vi "SSFG_sharp_Backup(Working).vi"() -> ()   [LabVIEW 2014]
uses:
  SSFG_States.ctl
  <vilib>/DAQmx/write.llb/DAQmx Write (Analog Wfm 1Chan NSamp).vi
  <vilib>/DAQmx/create/channels.llb/DAQmx Create Channel (AO-Voltage-Basic).vi
  <vilib>/DAQmx/configure/timing.llb/DAQmx Timing (Sample Clock).vi
  <vilib>/DAQmx/miscellaneous.llb/DAQmx Fill In Error Info.vi
  <resource>/objmgr/daqmx.rc
  <vilib>/measure/NI_MABase.lvlib
panel:
  in  "Attenuation":dbl
  out "Current State":string
  in  "Number of Samples/Cycle":dbl
  out "Waveform Graph":waveform(dbl)(graph)
  in  "stop":bool
  in  "Power Signal Parameters":T1={"Waveform Type"=0, "Amplitude"=1.0, "Frequency"=17.0} {"Frequency" format="%0.2p"; "Amplitude" scale=0.0..5.0; "Waveform Type" items=["Sine Wave", "Triangle Wave", "Square Wave", "Sawtooth Wave"]}
  out "Flicker":bool
  out "Swell":bool
  out "Sag":bool
  in  "Stop":bool
  in  "Update Rate":dbl=1000.0 format="%0.2f"
  in  "Physical Channel":tag
  in  "Flicker":T2
  in  "Swell":cluster{"Swell_Time (sec)":dbl, "Swell":bool}
  in  "Sag":cluster{"Sag_Time (sec)":dbl, "Sag":bool}
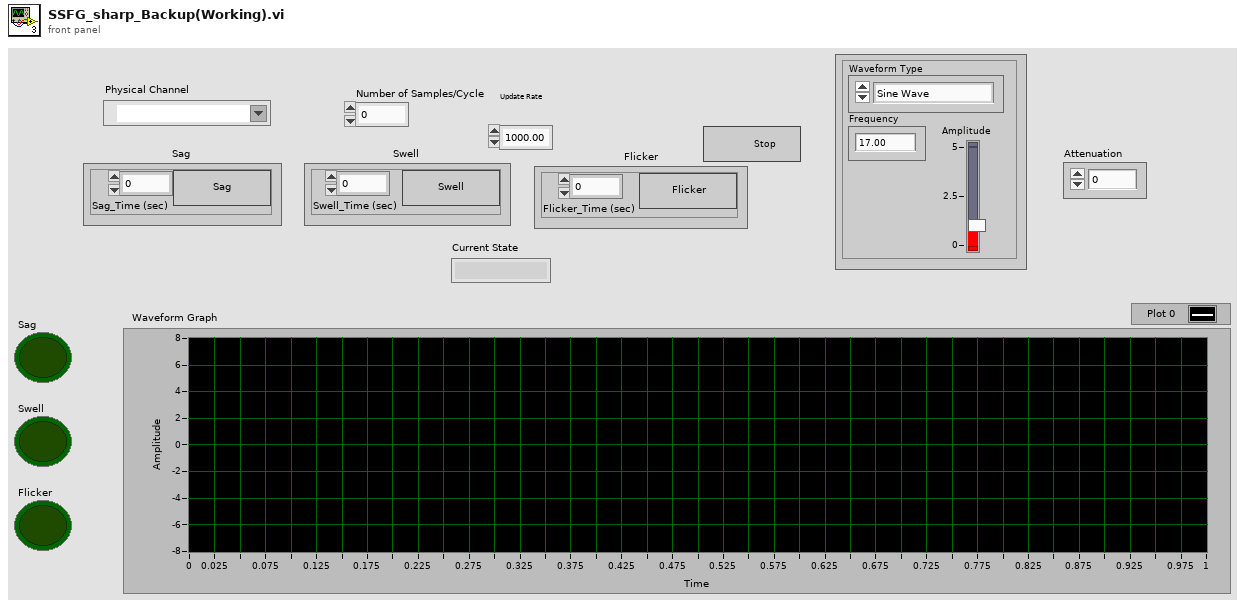
[diagram p1: front panel]
types:
  T1 = cluster{"Waveform Type":u16, "Amplitude":dbl, "Frequency":dbl}
  T2 = cluster{"Flicker_Time (sec)":dbl, "Flicker":bool}
  T3 = typedef "SSFG_States.ctl" = cluster{"State":string, "Disturbance_Time (sec)":dbl}
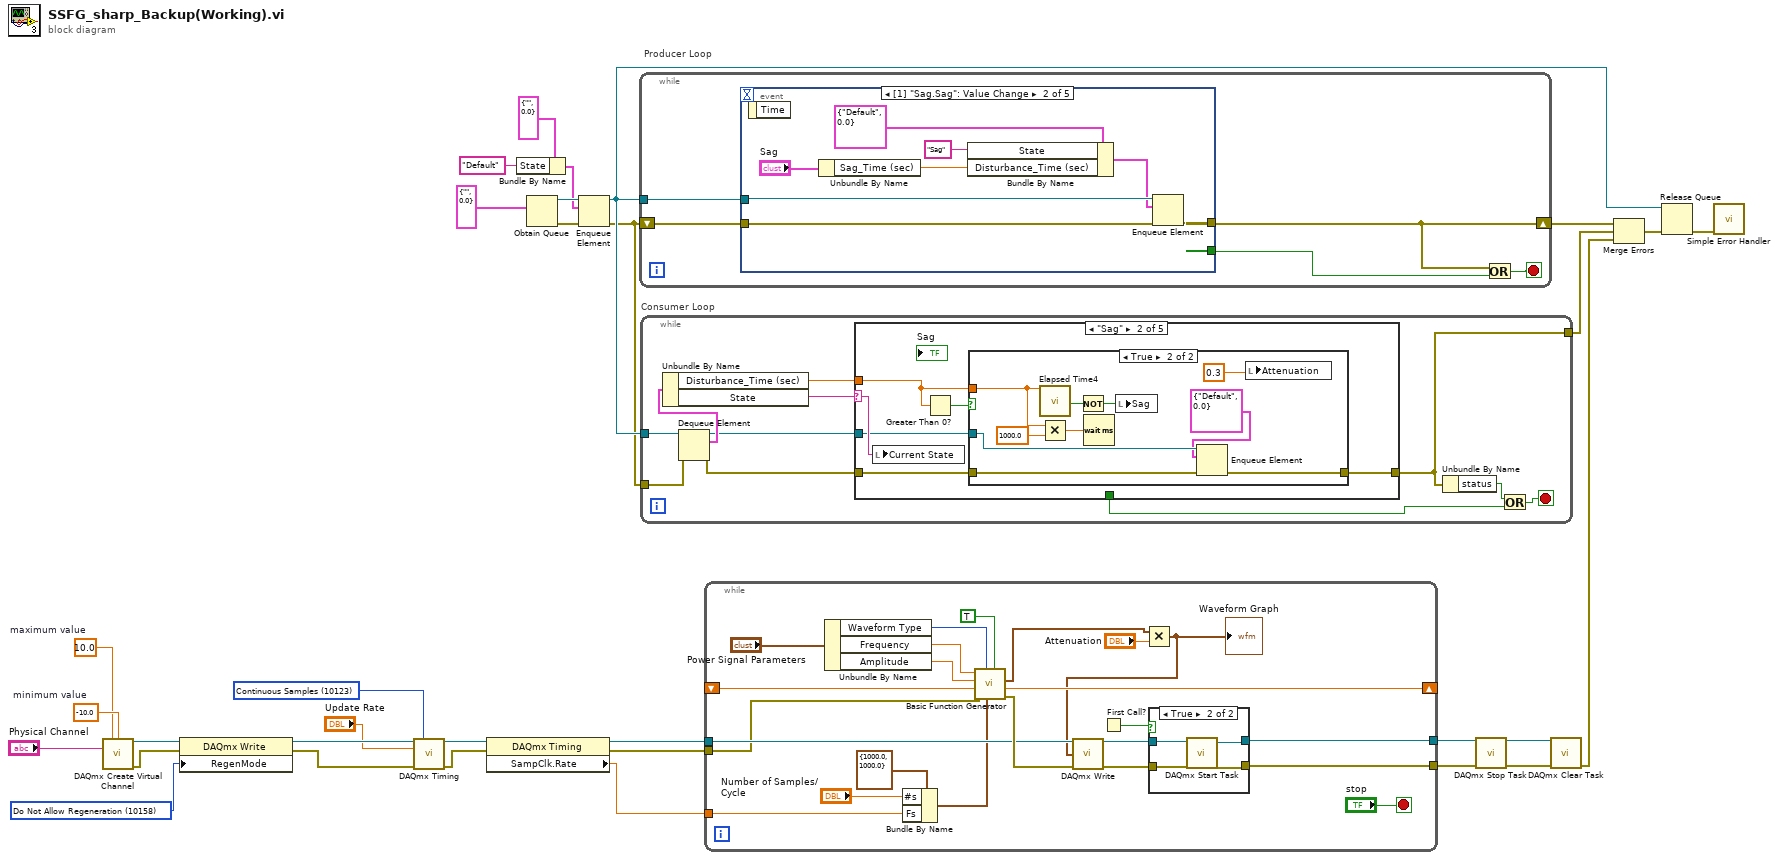
[diagram p0: block diagram]
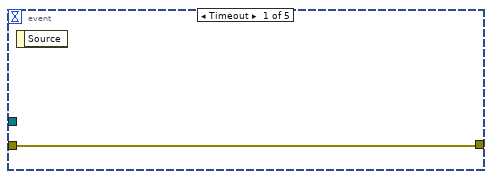
[diagram p2: hidden frame]
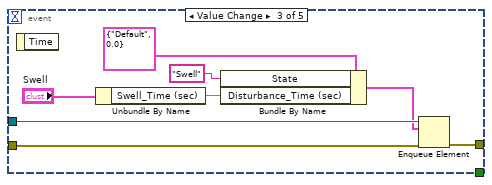
[diagram p3: hidden frame]
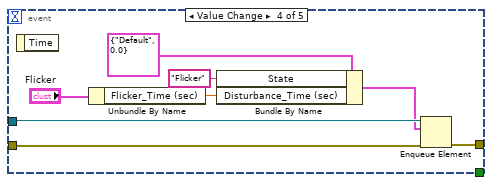
[diagram p4: hidden frame]
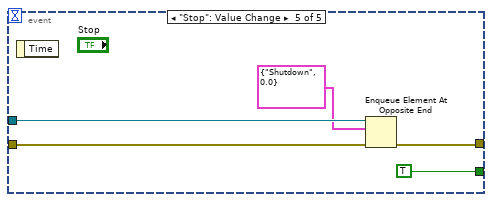
[diagram p5: hidden frame]
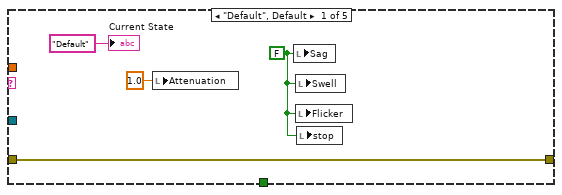
[diagram p6: hidden frame]
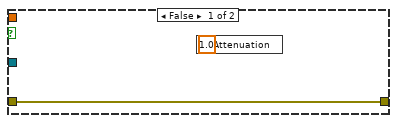
[diagram p7: hidden frame]
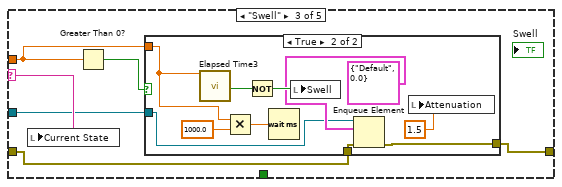
[diagram p8: hidden frame]
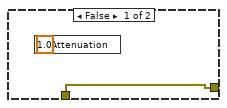
[diagram p9: hidden frame]
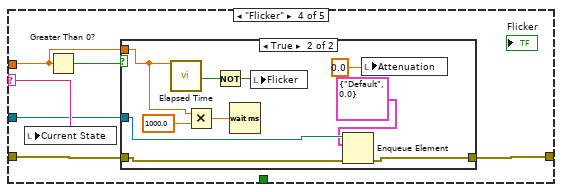
[diagram p10: hidden frame]
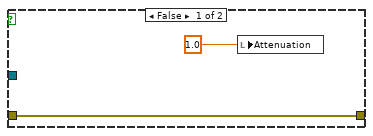
[diagram p11: hidden frame]
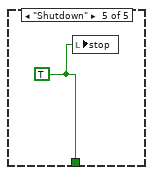
[diagram p12: hidden frame]
diagram:
  w14 = 10.0  # maximum value
  w15 = -10.0  # minimum value
  w26 = 10123 items=["Finite Samples"=10178, "Continuous Samples"=10123, "Hardware Timed Single Point"=12522] ("sample mode")
  w27 = 10158 items=["Allow Regeneration"=10097, "Do Not Allow Regeneration"=10158] ("RegenMode")
  n1 = call-poly <vilib>:"DAQmx Create Virtual Channel.vi"("maximum value"=w14, "minimum value"=w15, "physical channels"="Physical Channel") -> ("task out"=w31:refnum<k21>, "error out"=w29:errorcluster)  [unwired: 11 in]
  n2 = property class="DAQmx Write"(reference=w31, error in=w29, "RegenMode"=w27) -> (reference out=w30:refnum<k21>, error out=w28:errorcluster)
  n3 = call-poly <vilib>:"DAQmx Timing.vi"("task/channels in"=w30, "sample mode"=w26, "rate"="Update Rate", "error in"=w28) -> ("task out"=w24:refnum<k21>, "error out"=w23:errorcluster)  [unwired: 10 in]
  n4 = property class="DAQmx Timing"(reference=w24, error in=w23) -> (reference out=w20:refnum<k21>, error out=w21:errorcluster, "SampClk.Rate"=w19:dbl)
  n5 = Bundle By Name(cluster=T3 {"State"="", "Disturbance_Time (sec)"=0.0}, "State"="Default") -> (w6:T3)
  n6 = Obtain Queue(element data type=T3 {"State"="", "Disturbance_Time (sec)"=0.0}) -> (queue out=w10:refnum<queue>, error out=w9:errorcluster)  [unwired: 4 in, 1 out]
  n7 = Enqueue Element(queue=w10, element=w6, error in (no error)=w9) -> (queue out=w4:refnum<queue>, error out=w3:errorcluster)  [unwired: 1 in, 1 out]
  n8 = while "Producer Loop" {
    tunnel: w4 -> [w36]
    shift-right: [w34] -> w12
    shift-left: w3 -> [w35]
    stop <- w37 stop-if-true
    n9 = event shown="[1] \"Sag.Sag\": Value Change" {
      selector: _ -> [_ _ _ _ _]
      dyn-events: _ -> [_ _ _ _ _]
      timeout: _ -> [_ _ _ _ _]
      tunnel: w36 -> [_ w46 w54 w62 w67]
      tunnel: w35 -> [w38 w45 w53 w61 w66]
      tunnel: [w38 w44 w52 w60 w65] -> w34
      tunnel: [_ _ _ _ TRUE] -> w33
      event Timeout {
        n10 = event-data() -> ()  [unwired: 1 in, 1 out]
      }
      event "Sag.Sag": Value Change {
        n11 = event-data() -> ()  [unwired: 1 in, 1 out]
        n12 = Unbundle By Name("Sag") -> ("Sag_Time (sec)"=w41:dbl)
        n13 = Bundle By Name(cluster=T3 {"State"="Default", "Disturbance_Time (sec)"=0.0}, "State"="Sag", "Disturbance_Time (sec)"=w41) -> (w40:T3)
        n14 = Enqueue Element(queue=w46, element=w40, error in (no error)=w45) -> (error out=w44:errorcluster)  [unwired: 1 in, 2 out]
      }
      event "Swell.Swell": Value Change {
        n15 = event-data() -> ()  [unwired: 1 in, 1 out]
        n16 = Unbundle By Name("Swell") -> ("Swell_Time (sec)"=w50:dbl)
        n17 = Bundle By Name(cluster=T3 {"State"="Default", "Disturbance_Time (sec)"=0.0}, "State"="Swell", "Disturbance_Time (sec)"=w50) -> (w48:T3)
        n18 = Enqueue Element(queue=w54, element=w48, error in (no error)=w53) -> (error out=w52:errorcluster)  [unwired: 1 in, 2 out]
      }
      event "Flicker.Flicker": Value Change {
        n19 = event-data() -> ()  [unwired: 1 in, 1 out]
        n20 = Unbundle By Name("Flicker") -> ("Flicker_Time (sec)"=w57:dbl)
        n21 = Bundle By Name(cluster=T3 {"State"="Default", "Disturbance_Time (sec)"=0.0}, "State"="Flicker", "Disturbance_Time (sec)"=w57) -> (w56:T3)
        n22 = Enqueue Element(queue=w62, element=w56, error in (no error)=w61) -> (error out=w60:errorcluster)  [unwired: 1 in, 2 out]
      }
      event "Stop": Value Change {
        n23 = event-data() -> ()  [unwired: 1 in, 1 out]
        n24 = Enqueue Element At Opposite End(queue=w67, element=T3 {"State"="Shutdown", "Disturbance_Time (sec)"=0.0}, error in (no error)=w66) -> (error out=w65:errorcluster)  [unwired: 1 in, 2 out]
      }
    }
    n25 = Or(x=w34, y=w33) -> (x .or. y?=w37:bool)
  }
  n26 = while "Consumer Loop" {
    tunnel: [w71] -> w2
    tunnel: w4 -> [w76]
    tunnel: w3 -> [w75]
    stop <- w78 stop-if-true
    n27 = Dequeue Element(queue=w76, error in (no error)=w75) -> (queue out=w70:refnum<queue>, element=w74:T3, error out=w69:errorcluster)  [unwired: 1 in, 1 out]
    n28 = Unbundle By Name(w74) -> ("Disturbance_Time (sec)"=w68:dbl, "State"=w73:string)
    n29 = case shown="\"Sag\"" w73 {
      selector: w73 -> [_ w88 w106 w124 _]
      tunnel: [_ _ _ _ w137] -> w72
      tunnel: w69 -> [w81 w84 w103 w121 _]
      tunnel: [w81 w85 w102 w120 _] -> w71
      tunnel: w70 -> [_ w83 w101 w119 _]
      tunnel: w68 -> [_ w86 w104 w122 _]
      frame "Default", Default {
        w80 = FALSE ("Sag")
        n30 = local write "Attenuation"(1.0 ("Attenuation")) -> ()
        n31 = local write "Sag"(w80) -> ()
        n32 = local write "Swell"(w80) -> ()
        n33 = local write "Flicker"(w80) -> ()
        n34 = local write "stop"(w80) -> ()
        "Current State" <- "Default" ("Current State")
      }
      frame "Sag" {
        n35 = local write "Current State"(w88) -> ()
        n36 = Greater Than 0?(x=w86) -> (x > 0?=w87:bool)
        n37 = case shown="True" w87 {
          tunnel: w86 -> [_ w92]
          tunnel: [w89 w97] -> w85
          tunnel: w84 -> [w89 w96]
          tunnel: w83 -> [_ w95]
          frame False {
            n38 = local write "Attenuation"(1.0 ("y")) -> ()
          }
          frame True {
            n39 = call "Elapsed Time4"("Time Target (s)"=w92) -> ("Time has Elapsed"=w100:bool)  [unwired: 11 in, 7 out]
            n40 = Multiply(x=w92, y=1000.0) -> (x*y=w93:dbl)
            n41 = Not(x=w100) -> (.not. x?=w98:bool)
            n42 = Wait (ms)(milliseconds to wait=w93) -> ()  [unwired: 1 out]
            n43 = local write "Sag"(w98) -> ()
            n44 = Enqueue Element(queue=w95, element=T3 {"State"="Default", "Disturbance_Time (sec)"=0.0}, error in (no error)=w96) -> (error out=w97:errorcluster)  [unwired: 1 in, 2 out]
            n45 = local write "Attenuation"(0.3 ("y")) -> ()
          }
        }
      }
      frame "Swell" {
        n46 = local write "Current State"(w106) -> ()
        n47 = Greater Than 0?(x=w104) -> (x > 0?=w105:bool)
        n48 = case shown="True" w105 {
          tunnel: w104 -> [_ w111]
          tunnel: w103 -> [w107 w115]
          tunnel: [w107 w114] -> w102
          tunnel: w101 -> [_ w109]
          frame False {
            n49 = local write "Attenuation"(1.0 ("y")) -> ()
          }
          frame True {
            n50 = call "Elapsed Time3"("Time Target (s)"=w111) -> ("Time has Elapsed"=w117:bool)  [unwired: 11 in, 7 out]
            n51 = Multiply(x=w111, y=1000.0) -> (x*y=w113:dbl)
            n52 = Not(x=w117) -> (.not. x?=w118:bool)
            n53 = Wait (ms)(milliseconds to wait=w113) -> ()  [unwired: 1 out]
            n54 = local write "Swell"(w118) -> ()
            n55 = Enqueue Element(queue=w109, element=T3 {"State"="Default", "Disturbance_Time (sec)"=0.0}, error in (no error)=w115) -> (error out=w114:errorcluster)  [unwired: 1 in, 2 out]
            n56 = local write "Attenuation"(1.5 ("y")) -> ()
          }
        }
      }
      frame "Flicker" {
        n57 = local write "Current State"(w124) -> ()
        n58 = Greater Than 0?(x=w122) -> (x > 0?=w123:bool)
        n59 = case shown="True" w123 {
          tunnel: w122 -> [_ w128]
          tunnel: w121 -> [w125 w133]
          tunnel: [w125 w132] -> w120
          tunnel: w119 -> [_ w131]
          frame False {
            n60 = local write "Attenuation"(1.0 ("y")) -> ()
          }
          frame True {
            n61 = call "Elapsed Time"("Time Target (s)"=w128) -> ("Time has Elapsed"=w135:bool)  [unwired: 11 in, 7 out]
            n62 = Multiply(x=w128, y=1000.0) -> (x*y=w130:dbl)
            n63 = Not(x=w135) -> (.not. x?=w134:bool)
            n64 = Wait (ms)(milliseconds to wait=w130) -> ()  [unwired: 1 out]
            n65 = local write "Flicker"(w134) -> ()
            n66 = Enqueue Element(queue=w131, element=T3 {"State"="Default", "Disturbance_Time (sec)"=0.0}, error in (no error)=w133) -> (error out=w132:errorcluster)  [unwired: 1 in, 2 out]
            n67 = local write "Attenuation"(0.0 ("y")) -> ()
          }
        }
      }
      frame "Shutdown" {
        w137 = TRUE
        n68 = local write "stop"(w137) -> ()
      }
    }
    n69 = Unbundle By Name(w71) -> ("status"=w77:bool)
    n70 = Or(x=w77, y=w72) -> (x .or. y?=w78:bool)
  }
  n71 = while {
    tunnel: [w150] -> w18
    tunnel: [w149] -> w22
    tunnel: w20 -> [w148]
    tunnel: w21 -> [w147]
    tunnel: w19 -> [w144]
    shift-right: [w141] -> _
    shift-left: _ -> [w140]
    stop <- "stop" stop-if-true
    n72 = Unbundle By Name("Power Signal Parameters") -> ("Waveform Type"=w155:u16, "Frequency"=w154:dbl, "Amplitude"=w153:dbl)
    n73 = Bundle By Name(cluster=cluster{"Fs":dbl, "#s":dbl} {"Fs"=1000.0, "#s"=1000.0} ("sampling info"), "#s"="Number of Samples/Cycle", "Fs"=w144) -> (w146:cluster{"Fs":dbl, "#s":dbl})
    n74 = call <vilib>:"Basic Function Generator.vi"("reset signal"=TRUE, "sampling info"=w146, "signal type"=w155, "error in (no error)"=w147, "phase"=w140, "amplitude"=w153, "frequency"=w154) -> ("error out"=w157:errorcluster, "phase out"=w141:dbl, "signal out"=w142:waveform(dbl))  [unwired: 2 in]
    n75 = First Call?() -> (First Call?: T/F=w156:bool)
    n76 = Multiply(x=w142, y="Attenuation") -> (x*y=w139:waveform(dbl))
    "Waveform Graph" <- w139
    n77 = call-poly <vilib>:"DAQmx Write.vi"("task/channels in"=w148, "data"=w139, "error in"=w157) -> ("task out"=w159:refnum<k21>, "error out"=w158:errorcluster)  [unwired: 10 in, 1 out]
    n78 = case shown="True" w156 {
      tunnel: w159 -> [w161 w166]
      tunnel: w158 -> [w162 w165]
      tunnel: [w161 w164] -> w149
      tunnel: [w162 w163] -> w150
      frame False {
      }
      frame True {
        n79 = call <vilib>:"DAQmx Start Task.vi"("task/channels in"=w166, "error in"=w165) -> ("task out"=w164:refnum<k21>, "error out"=w163:errorcluster)  [unwired: 12 in]
      }
    }
  }
  n80 = call <vilib>:"DAQmx Stop Task.vi"("task/channels in"=w22, "error in"=w18) -> ("task out"=w17:refnum<k21>, "error out"=w16:errorcluster)  [unwired: 12 in]
  n81 = call <vilib>:"DAQmx Clear Task.vi"("task in"=w17, "error in"=w16) -> ("error out"=w1:errorcluster)  [unwired: 13 in]
  n82 = Merge Errors(w12, w2, w1) -> (w11:errorcluster)
  n83 = Release Queue(queue=w4, error in (no error)=w11) -> (error out=w13:errorcluster)  [unwired: 1 in, 2 out]
  n84 = call <vilib>:"Simple Error Handler.vi"("error in (no error)"=w13) -> ()  [unwired: 4 in, 5 out]
